vi "FOCUS_V42.vi"(9 "X-pixels":sgl=256.0, 11 "Run":bool) -> (0 "Retrace pixels":sgl, 10 "Pixel Clock (Hz)":sgl)   [LabVIEW 2010] (continued)
            n1000 = Array Max & Min(array=w3024) -> (max value=w3028:dbl, min value=w3027:dbl)  [unwired: 2 out]
            n1001 = Greater?(x=w3028, y=w3021) -> (0:w3026:bool)
            n1002 = Less?(x=w3027, y=w3022) -> (x < y?=w3025:bool)
            n1003 = Or(x=w3026, y=w3025) -> (x .or. y?=w3023:bool)
            n1004 = case shown="False" w3023 {
              tunnel: [u32 16711680 u32 0] -> w3029
              frame True {
              }
              frame False {
                (unwired) u32 16756736
              }
            }
          }
        }
        n1005 = Bundle(w2039, w2040) -> (→"Galvos":cluster{dbl[], dbl[]})  [unwired: 1 in]
        n1006 = local read "frame/line indicator"() -> (w2024:u16)
        n1007 = local read "frame/line indicator"() -> (w1884:u16)
        n1008 = property class="DAQmx Buffer"(reference=w1951, error in=w1949, "Input:Buffer Size"=u32 10000000 ("Input.BufSize")) -> (reference out=w1950:refnum<k21>, error out=w1948:errorcluster)
        n1009 = Concatenate Strings(w1896, tag "/PXI_Trig2" ("source terminal")) -> (w1988:string)
        n1010 = call-poly <vilib>:"DAQmx Create Channel (CO-Pulse Generation-Ticks).vi"("high ticks"=w1876, "low ticks"=w1874, "counter"=w1934, "source of ticks"=w1928, "error in"=w1923, "initial delay"=w1877) -> ("task out"=w1960:refnum<k21>, "error out"=w1959:errorcluster)  [unwired: 8 in]
        n1011 = Greater Or Equal?(x=w2024, y=3.0) -> (x >= y?=w2023:bool)
        n1012 = Concatenate Strings(w1896, tag "/PXI_Trig2" ("destination terminal")) -> (w1992:string)
        n1013 = Bundle("Trigger?"="Trigger?", "Type"="Type", "Level [V]"="Level [V]", "slope"="slope") -> (w1907:T17)  [unwired: 1 in]
        n1014 = Type Cast(type=tag "" ("destination terminal"), x=w1988) -> (*(type *) &x=w1985:tag)
        n1015 = Concatenate Strings(w1896, tag "/10MHzRefClock" ("source terminal")) -> (w1997:string)
        n1016 = Type Cast(type=tag "" ("destination terminal"), x=w1992) -> (*(type *) &x=w1989:tag)
        n1017 = Type Cast(type=tag "" ("destination terminal"), x=w1997) -> (*(type *) &x=w1994:tag)
        n1018 = call-poly <vilib>:"DAQmx Timing (Implicit).vi"("task/channels in"=w1960, "sample mode"=w1958, "error in"=w1959) -> ("task out"=w1957:refnum<k21>, "error out"=w1956:errorcluster)  [unwired: 11 in]
        n1019 = case shown="3" w1884 {
          tunnel: [_ _ w3014 w3017 w3018] -> w2029
          frame 0, Default {
          }
          frame 1 {
          }
          frame 2 {
            n1020 = local read "Y-lines"() -> (w3015:sgl)
            n1021 = local read "Number of frames"() -> (w3016:sgl)
            n1022 = Multiply(x=w3015, y=w3016) -> (x*y=w3014:sgl)
          }
          frame 3 {
            n1023 = local read "Y-lines FreeLine"() -> (w3017:sgl)
          }
          frame 4 {
            n1024 = local read "Y-lines FreeLine"() -> (w3018:sgl)
          }
        }
        n1025 = local read "Fiberscope\nMode"() -> (w1893:bool)
        n1026 = case shown="False" w1893 {
          tunnel: w2023 -> [w2080 _]
          tunnel: w1946 -> [w2079 _]
          tunnel: [w2078 w2083] -> w1915
          frame False {
            n1027 = case shown="False" w2080 {
              tunnel: [w2081 w2082] -> w2078
              tunnel: w2079 -> [_ _]
              frame False {
                n1028 = local read "Pixel Clock (Hz)"() -> (w2081:sgl)
              }
              frame True {
                n1029 = local read "Pixel Clock (Hz) FreeLine"() -> (w2082:sgl)
              }
            }
          }
          frame True {
            n1030 = local read "Pixel Clock (Hz) FScope"() -> (w2083:sgl)
          }
        }
        n1031 = case shown="True" w1916 {
          tunnel: [_ w2977] -> w2013
          tunnel: [_ w2976] -> w2012
          tunnel: w1915 -> [_ w2973]
          tunnel: w1921 -> [_ w2961]
          frame False {
          }
          frame True {
            w2980 = 10123 items=["Finite Samples"=10178, "Continuous Samples"=10123, "Hardware Timed Single Point"=12522] ("sample mode")
            w2981 = 10171 items=["Rising"=10280, "Falling"=10171] ("edge")
            n1032 = local read "AI Device"() -> (w2948:tag)
            n1033 = Concatenate Strings(w2948, tag "/ai0," ("physical channels"), w2948, tag "/ai1," ("physical channels"), w2948, tag "/ai2," ("physical channels"), w2948, tag "/ai3" ("physical channels")) -> (w2970:string)
            n1034 = Type Cast(type=tag "" ("physical channels"), x=w2970) -> (*(type *) &x=w2967:tag)
            n1035 = local read "AO/DIO Device"() -> (w2951:tag)
            n1036 = call-poly <vilib>:"DAQmx Create Channel (AI-Voltage-Basic).vi"("maximum value"=10.0, "physical channels"=w2967, "error in"=w2961) -> ("task out"=w2978:refnum<k21>, "error out"=w2979:errorcluster)  [unwired: 11 in]
            n1037 = Concatenate Strings(tag "/" ("destination terminal"), w2951, tag "/ao/SampleClock" ("source")) -> (w2952:string)
            n1038 = Type Cast(type=tag "" ("source"), x=w2952) -> (*(type *) &x=w2950:tag)
            n1039 = call-poly <vilib>:"DAQmx Timing (Sample Clock).vi"("task/channels in"=w2978, "sample mode"=w2980, "rate"=w2973, "source"=w2950, "error in"=w2979) -> ("task out"=w2960:refnum<k21>, "error out"=w2959:errorcluster)  [unwired: 9 in]
            n1040 = property class="DAQmx Buffer"(reference=w2960, error in=w2959, "Input:Buffer Size"=u32 5000000 ("Input.BufSize")) -> (reference out=w2957:refnum<k21>, error out=w2958:errorcluster)
            n1041 = Concatenate Strings(tag "/" ("destination terminal"), w2951, tag "/ao/StartTrigger" ("source")) -> (w2966:string)
            n1042 = Type Cast(type=tag "" ("source"), x=w2966) -> (*(type *) &x=w2964:tag)
            n1043 = call-poly <vilib>:"DAQmx Start Trigger (Digital Edge).vi"("task/channels in"=w2957, "source"=w2964, "edge"=w2981, "error in"=w2958) -> ("task out"=w2975:refnum<k21>, "error out"=w2974:errorcluster)  [unwired: 10 in]
            n1044 = call <vilib>:"DAQmx Start Task.vi"("task/channels in"=w2975, "error in"=w2974) -> ("task out"=w2977:refnum<k21>, "error out"=w2976:errorcluster)  [unwired: 12 in]
          }
        }
        n1045 = call "AOConfigwriteDAQmx.vi"("AO.UseOnlyOnBrdMem"=FALSE, "TriggerCluster"=w1907, "Trigger Source"=w1906, "Sampling"=w1914, "rate"=w1915, "data"=w1888, "error in"=w1921, "RegenMode"=w2026, "Output.OnbrdBufSize"=w1946, "physical channels"=w2014) -> ("error out"=w2008:errorcluster, "task out"=w2007:refnum<k21>)
        n1046 = call <vilib>:"DAQmx Connect Terminals.vi"("source terminal"=w1994, "destination terminal"=w1989, "error in"=w2008) -> ("error out"=w2027:errorcluster)  [unwired: 12 in]
        n1047 = Concatenate Strings(w1896, tag "/ao/StartTrigger" ("source terminal")) -> (w1899:string)
        n1048 = call <vilib>:"DAQmx Start Task.vi"("task/channels in"=w1957, "error in"=w1956) -> ("task out"=w1955:refnum<k21>, "error out"=w1922:errorcluster)  [unwired: 12 in]
        n1049 = call-poly <vilib>:"DAQmx Timing (Sample Clock).vi"("task/channels in"=w1950, "sample mode"=w2011, "rate"=w1915, "source"=w1963, "error in"=w1948) -> ("task out"=w2010:refnum<k21>, "error out"=w2009:errorcluster)  [unwired: 9 in]
        n1050 = Concatenate Strings(w1896, tag "/PFI2" ("destination terminal")) -> (w1984:string)
        n1051 = Type Cast(type=tag "" ("destination terminal"), x=w1899) -> (*(type *) &x=w1895:tag)
        n1052 = Concatenate Strings(w1896, tag "/PFI5" ("destination terminal")) -> (w1976:string)
        n1053 = Concatenate Strings(w1896, tag "/PFI7" ("destination terminal")) -> (w1905:string)
        n1054 = local read "frame/line indicator"() -> (w2037:u16)
        n1055 = Type Cast(type=tag "" ("destination terminal"), x=w1984) -> (*(type *) &x=w1981:tag)
        n1056 = call <vilib>:"DAQmx Connect Terminals.vi"("source terminal"=w1985, "destination terminal"=w1981, "error in"=w2027) -> ("error out"=w1902:errorcluster)  [unwired: 12 in]
        n1057 = property on="Galvos" class="XYGraph (strict)"("Plot Area:Colors:FG Color"=w2041, "Plot Area:Colors:BG Color"=w2041) -> ()  [unwired: 2 in, 2 out]
        n1058 = Concatenate Strings(w1896, tag "/ao/SampleClock" ("source terminal")) -> (w1980:string)
        n1059 = Type Cast(type=tag "" ("destination terminal"), x=w1976) -> (*(type *) &x=w1973:tag)
        n1060 = Type Cast(type=tag "" ("destination terminal"), x=w1905) -> (*(type *) &x=w1900:tag)
        n1061 = call <vilib>:"DAQmx Connect Terminals.vi"("source terminal"=w1895, "destination terminal"=w1900, "error in"=w1902) -> ("error out"=w1901:errorcluster)  [unwired: 12 in]
        n1062 = call <vilib>:"DAQmx Start Task.vi"("task/channels in"=w2010, "error in"=w2009) -> ("task out"=w2016:refnum<k21>, "error out"=w2015:errorcluster)  [unwired: 12 in]
        n1063 = for {
          N: w2029 -> [_]
          tunnel: [w3019] -> w2030 mode=indexing
          i -> [w3019]
        }
        n1064 = Type Cast(type=tag "" ("destination terminal"), x=w1980) -> (*(type *) &x=w1977:tag)
        n1065 = call <vilib>:"DAQmx Connect Terminals.vi"("source terminal"=w1977, "destination terminal"=w1973, "error in"=w1901) -> ()  [unwired: 12 in, 1 out]
      }
    }
    n1066 = local read "Image3Array"() -> (w170:u8[][])
    n1067 = local read "Image4Array"() -> (w186:u8[][])
    n1068 = local read "Image1Array"() -> (w175:u8[][])
    n1069 = local read "Image2Array"() -> (w185:u8[][])
    n1070 = flat-sequence {
      tunnel: w175 -> [_]
      frame #0 {
        n1071 = property on="Property Node" class="VI"() -> ("VI Path"=w329:path)  [unwired: 2 in, 2 out]
        n1072 = Initialize Array(u8 0 ("x 2")) -> (w314:u8[])  [unwired: 1 in]
        n1073 = Strip Path(path=w329) -> (stripped path=w305:path)  [unwired: 1 out]
        n1074 = local read "VISA Sutter MP-285"() -> (w320:refnum<visa-resource-name>)
        n1075 = local read "MaiTai setting Path"() -> (w316:path)
        n1076 = local read "VISA XPG-ADC"() -> (w318:refnum<visa-resource-name>)
        n1077 = Strip Path(path=w305) -> ()  [unwired: 2 out]
        n1078 = local read "AO/DIO Device"() -> (w333:tag)
        n1079 = local read "AI Device"() -> (w326:tag)
        n1080 = Build Path(base path=w305, name or relative path="FOCUS.cfg") -> (appended path=w309:path)
        n1081 = Path To String(path=w316) -> (string=w315:string)
        n1082 = Type Cast(type="" ("name or relative path"), x=w318) -> (*(type *) &x=w317:string)
        n1083 = Type Cast(type="" ("name or relative path"), x=w320) -> (*(type *) &x=w319:string)
        n1084 = Type Cast(type=w314, x=w326) -> (*(type *) &x=w300:u8[])
        n1085 = Type Cast(type=w314, x=w315) -> (*(type *) &x=w313:u8[])
        n1086 = Type Cast(type=w314, x=w317) -> (*(type *) &x=w323:u8[])
        n1087 = Type Cast(type=w314, x=w319) -> (*(type *) &x=w324:u8[])
        n1088 = Type Cast(type=w314, x=w333) -> (*(type *) &x=w304:u8[])
        n1089 = Array Size(array=w300) -> (size(s)=w301:i32)
        n1090 = Array Size(array=w313) -> (size(s)=w312:i32)
        n1091 = Array Size(array=w304) -> (size(s)=w303:i32)
        n1092 = To Unsigned Byte Integer(number=w301) -> (unsigned 8bit integer=w299:u8)
        n1093 = To Unsigned Byte Integer(number=w312) -> (unsigned 8bit integer=w311:u8)
        n1094 = call <vilib>:"Open_Create_Replace File.vi"("advisory dialog? (display:T)"=FALSE, "function (open:0)"=T8."create or replace", "file path"=w309) -> ("error out"=w307:errorcluster, "refnum"=w308:refnum<file>)  [unwired: 5 in, 2 out]
        n1095 = To Unsigned Byte Integer(number=w303) -> (unsigned 8bit integer=w302:u8)
        n1096 = Build Array (concatenate)(w302, w304, w299, w300, w324, w323, w311, w313) -> (w325:u8[])
        n1097 = Write to Binary File(file (use dialog)=w308, data=w325, error in=w307, 5:FALSE ("prepend array or string size? (T)")) -> (refnum out=w327:refnum<file>, error out=w328:errorcluster)  [unwired: 2 in, 1 out]
        n1098 = Close File(refnum=w327, error in=w328) -> (error out=w331:errorcluster)  [unwired: 1 out]
        n1099 = call <vilib>:"Simple Error Handler.vi"("error in (no error)"=w331) -> ()  [unwired: 4 in, 5 out]
      }
    }
    n1100 = Equal?(x=w181, y=u16 4) -> (x = y?=w179:bool)
    n1101 = local read "ScanLineFreeLine"() -> (w197:sgl[][])
    n1102 = Index Array(array=w197, index (row)=0 ("disabled index (col)")) -> (element=w196:sgl[])  [unwired: 1 in]
    n1103 = Index Array(array=w197, index (row)=1 ("disabled index (col)")) -> (element=w177:sgl[])  [unwired: 1 in]
    n1104 = case shown="False" w179 {
      tunnel: [w334 w338] -> w178
      tunnel: w177 -> [w335 _]
      frame False {
        n1105 = Array Size(array=w335) -> (size(s)=w336:i32)
        n1106 = Initialize Array(sgl 0.0 ("element"), w336) -> (w334:sgl[])
      }
      frame True {
        n1107 = local read "Zsin3D"() -> (w338:sgl[])
      }
    }
    n1108 = Greater Or Equal?(x=w181, y=u16 3) -> (x >= y?=w182:bool)
    n1109 = local write "Ready?"(FALSE ("Ready?")) -> ()
    n1110 = property on="Image 2" class="IntGraph (strict)"() -> ("Color Table"=w288:u32[])  [unwired: 2 in, 2 out]
    n1111 = Interleave 1D Arrays(w196, w177, w178) -> (w192:sgl[])
    n1112 = local read "Positions"() -> (w191:sgl[])
    n1113 = local read "Focus"() -> (w207:bool)
    n1114 = local write "OpenShutter"(FALSE ("OpenShutter")) -> ()
    n1115 = local read "Channel selector"() -> (w159:u8)
    n1116 = Array Size(array=w192) -> (size(s)=w193:i32)
    n1117 = local write "Run"(w207) -> ()
    n1118 = Build Array (concatenate)(w193, w192, w191) -> (w184:sgl[])
    n1119 = flat-sequence {
      tunnel: [w430] -> w295
      tunnel: [w429] -> w162
      tunnel: [w397] -> w291
      tunnel: [w398] -> w290
      tunnel: w288 -> [w408]
      tunnel: w258 -> [w425]
      tunnel: w287 -> [w424]
      tunnel: [w423] -> w286
      tunnel: [w422] -> w285
      tunnel: w282 -> [w421]
      tunnel: w281 -> [w420]
      tunnel: [w399] -> w276
      tunnel: [w400] -> w275
      tunnel: [w386] -> w263
      tunnel: [w403] -> w218
      tunnel: [w402] -> w217
      tunnel: [w401] -> w209
      tunnel: w206 -> [w380]
      tunnel: w170 -> [w379]
      tunnel: w186 -> [w378]
      tunnel: w175 -> [w377]
      tunnel: w185 -> [w376]
      tunnel: w184 -> [w375]
      tunnel: w182 -> [w374]
      tunnel: w167 -> [w362]
      tunnel: [w362] -> w166
      tunnel: [w356] -> w160
      tunnel: w159 -> [w355]
      frame #0 {
        w407 = FALSE ("data")
        w419 = i8 -1 ("element")
        n1120 = local read "Mode selector"() -> (w371:u16)
        n1121 = local read "frame/line indicator"() -> (w427:u16)
        n1122 = local read "ImageSelector"() -> (w416:bool)
        n1123 = Split Number(x=w408) -> (lo(x)=w410:u16[])  [unwired: 1 out]
        n1124 = Split Number(x=w410) -> (lo(x)=w409:u8[])  [unwired: 1 out]
        n1125 = Equal?(x=w427, y=4) -> (x = y?=w361:bool)
        n1126 = Equal?(x=w371, y=4) -> (x = y?=w358:bool)
        n1127 = Or(x=w361, y=w362) -> (x .or. y?=w360:bool)
        n1128 = property on="Intensity" class="Slide (strict)"("Scale.Range:Maximum"="IntensityScaleMax") -> ()  [unwired: 2 in, 2 out]
        n1129 = Not(x=w358) -> (.not. x?=w359:bool)
        n1130 = And(x=w359, y=w360) -> (x .and. y?=w357:bool)
        n1131 = case shown="False" w357 {
          tunnel: [w455 _] -> w395
          tunnel: [w454 _] -> w396
          tunnel: w358 -> [w453 _]
          frame False {
            n1132 = case shown="True" w453 {
              tunnel: [w465 w478] -> w455
              tunnel: [w464 w477] -> w454
              frame False {
                n1133 = local read "AO/DIO Device"() -> (w461:tag)
                n1134 = Concatenate Strings(w461, tag "/ao3" ("physical channels")) -> (w459:string)
                n1135 = Type Cast(type=tag "" ("physical channels"), x=w459) -> (*(type *) &x=w457:tag)
                n1136 = call-poly <vilib>:"DAQmx Create Channel (AO-Voltage-Basic).vi"("physical channels"=w457) -> ("task out"=w462:refnum<k21>, "error out"=w463:errorcluster)  [unwired: 13 in]
                n1137 = local read "Intensity"() -> (w456:sgl)
                n1138 = call-poly <vilib>:"DAQmx Write (Analog DBL 1Chan 1Samp).vi"("task/channels in"=w462, "data"=w456, "error in"=w463) -> ("task out"=w465:refnum<k21>, "error out"=w464:errorcluster)  [unwired: 10 in, 1 out]
              }
              frame True {
                n1139 = local read "AO/DIO Device"() -> (w466:tag)
                n1140 = Concatenate Strings(w466, tag "/ao2," ("physical channels"), w466, tag "/ao3" ("physical channels")) -> (w473:string)
                n1141 = Type Cast(type=tag "" ("physical channels"), x=w473) -> (*(type *) &x=w471:tag)
                n1142 = call-poly <vilib>:"DAQmx Create Channel (AO-Voltage-Basic).vi"("physical channels"=w471) -> ("task out"=w475:refnum<k21>, "error out"=w476:errorcluster)  [unwired: 13 in]
                n1143 = local read "Intensity"() -> (w469:sgl)
                n1144 = Build Array(sgl 0.0 ("element"), w469) -> (w468:sgl[])
                n1145 = call-poly <vilib>:"DAQmx Write (Analog 1D DBL NChan 1Samp).vi"("task/channels in"=w475, "data"=w468, "error in"=w476) -> ("task out"=w478:refnum<k21>, "error out"=w477:errorcluster)  [unwired: 10 in, 1 out]
              }
            }
          }
          frame True {
          }
        }
        n1146 = local read "Fiberscope\nMode"() -> (w401:bool)
        n1147 = call "VISA MP-285 GetSet Speed.vi"("Input: Duty Cluster"=w380, "Input: Speed in microns/sec"="Sutter Speed [um/s]") -> ("Output: Duty Cluster"=w390:T18)  [unwired: 1 out]
        n1148 = call "VISA MP-285 Get Position.vi"("Input: Duty Cluster"=w390) -> ("Output: X axis (microns)"=w382:dbl, "Output: Y axis (microns)"=w383:dbl, "Output: Z axis (microns)"=w388:dbl, "Output: Duty Cluster"=w387:T18)
        n1149 = Multiply(x=w382, y="Sutter scale x") -> (x*y=→"x-positionstart (um)":dbl)
        n1150 = Multiply(x=w383, y="Sutter scale y") -> (x*y=→"y-positionstart (um)":dbl)
        n1151 = local read "frame scan finished?"() -> (w370:bool)
        n1152 = Multiply(x="Sutter scale z", y=w388) -> (x*y=w381:dbl)
        "z-positionstart (um)" <- w381
        n1153 = local read "AO/DIO Device"() -> (w413:tag)
        n1154 = property on="ImageSlide" class="Slide (strict)"() -> ("Scale.Range:Maximum"=w418:dbl, "Visible"=w417:bool)  [unwired: 2 in, 2 out]
        n1155 = case shown="True" w401 {
          tunnel: [_ w447] -> w403
          tunnel: [_ w446] -> w402
          frame False {
          }
          frame True {
            w441 = TRUE ("element")
            n1156 = local read "AO/DIO Device"() -> (w443:tag)
            n1157 = Concatenate Strings(w443, tag "/port2/line6," ("lines"), w443, tag "/port2/line7" ("lines")) -> (w452:string)
            n1158 = Type Cast(type=tag "" ("lines"), x=w452) -> (*(type *) &x=w450:tag)
            n1159 = call-poly <vilib>:"DAQmx Create Channel (DO-Digital Output).vi"("lines"=w450) -> ("task out"=w449:refnum<k21>, "error out"=w448:errorcluster)  [unwired: 13 in]
            n1160 = Build Array(w441, w441) -> (w442:bool[])
            n1161 = call-poly <vilib>:"DAQmx Write (Digital 1D Bool 1Chan 1Samp).vi"("task/channels in"=w449, "data"=w442, "error in"=w448) -> ("task out"=w447:refnum<k21>, "error out"=w446:errorcluster)  [unwired: 10 in, 1 out]
          }
        }
        n1162 = Concatenate Strings(w413, tag "/port1/line1" ("lines")) -> (w415:string)
        n1163 = local read "GetFirst"() -> (w384:bool)
        n1164 = local read "GetLast"() -> (w385:bool)
        n1165 = Type Cast(type=tag "" ("lines"), x=w415) -> (*(type *) &x=w411:tag)
        n1166 = And(x=w370, y="Go back?") -> (x .and. y?=w368:bool)
        n1167 = And(x=w384, y=w385) -> (x .and. y?=w373:bool)
        n1168 = call-poly <vilib>:"DAQmx Create Channel (DO-Digital Output).vi"("lines"=w411) -> ("task out"=w406:refnum<k21>, "error out"=w405:errorcluster)  [unwired: 13 in]
        "Shutter" <- w406
        n1169 = Or(x=w368, y=w373) -> (x .or. y?=w366:bool)
        n1170 = case shown="True" w366 {
          tunnel: w387 -> [w432 w440]
          tunnel: [w432 w439] -> w386
          tunnel: w381 -> [_ w437]
          tunnel: [FALSE ("IntDevUsed 2") FALSE ("IntDevUsed 2")] -> w367
          frame False {
          }
          frame True {
            n1171 = local read "FirstPosition"() -> (w436:sgl)
            n1172 = local read "Sutter scale z"() -> (w433:sgl)
            n1173 = Subtract(x=w436, y=w437) -> (x-y=w435:dbl)
            n1174 = Divide(x=w435, y=w433) -> (x/y=w438:dbl)
            n1175 = call "VISA MP-285 Step.vi"("Input: Duty Cluster"=w440, "Input: Delta Z axis (microns)"=w438) -> ("Output: Duty Cluster"=w439:T18)  [unwired: 2 in, 3 out]
          }
        }
        n1176 = local write "frame scan finished?"(w367) -> ()
        n1177 = local write "Shutter open"(w407) -> ()
        n1178 = call-poly <vilib>:"DAQmx Write (Digital Bool 1Line 1Point).vi"("task/channels in"=w406, "data"=w407, "error in"=w405) -> ("task out"=w393:refnum<k21>, "error out"=w394:errorcluster)  [unwired: 10 in, 1 out]
        n1179 = while {
          tunnel: ["Run"] -> w430
          tunnel: ["End experiment"] -> w429
          shift-right: [w580] -> _
          shift-left: w408 -> [w583]
          shift-right: [w578] -> _
          shift-left: FALSE ("Visible") -> [w579]
          tunnel: w425 -> [w577]
          tunnel: w424 -> [w576]
          tunnel: [w577] -> w423
          tunnel: [w576] -> w422
          tunnel: w421 -> [w574]
          tunnel: w420 -> [w566]
          shift-right: [w539] -> _
          shift-left: w419 -> [w540]
          shift-right: [w537] -> _
          shift-left: w419 -> [w538]
          tunnel: w418 -> [w536]
          tunnel: w417 -> [w535]
          shift-right: [w528] -> _
          shift-left: w416 -> [w527]
          shift-right: [w521] -> _
          shift-left: w409 -> [w522]
          tunnel: [w501] -> w400
          tunnel: [w500] -> w399
          tunnel: [w505] -> w398
          tunnel: [w504] -> w397
          tunnel: w396 -> [w507]
          tunnel: w395 -> [w506]
          tunnel: w394 -> [w503]
          tunnel: w393 -> [w502]
          tunnel: w379 -> [w487]
          tunnel: w378 -> [w486]
          tunnel: w377 -> [w488]
          tunnel: w376 -> [w489]
          tunnel: w375 -> [w492]
          tunnel: w374 -> [w490]
          tunnel: [w480] -> w356
          shift-right: [w479] -> _
          shift-left: w355 -> [w481]
          i -> [w526]
          stop <- w517 stop-if-true
          n1180 = local read "index (row)1"() -> (w545:i32)
          n1181 = property on="Image 2" class="IntGraph (strict)"() -> ("Color Table"=w582:u32[])  [unwired: 2 in, 2 out]
          n1182 = event shown="[0] Timeout" {
            selector: _ -> [_ _ _ _ _ _ _ _ _ _ _ _ _ _ _ _ _ _ _ _ _ _ _ _ _ _ _ _ _ _ _ _ _ _ _]
            dyn-events: _ -> [_ _ _ _ _ _ _ _ _ _ _ _ _ _ _ _ _ _ _ _ _ _ _ _ _ _ _ _ _ _ _ _ _ _ _]
            timeout: 0 -> [_ _ _ _ _ _ _ _ _ _ _ _ _ _ _ _ _ _ _ _ _ _ _ _ _ _ _ _ _ _ _ _ _ _ _]
            tunnel: [FALSE ("Fiberscope\nMode") TRUE ("Fiberscope\nMode") TRUE ("Fiberscope\nMode") TRUE ("Fiberscope\nMode") TRUE ("Fiberscope\nMode") TRUE ("Fiberscope\nMode") TRUE ("Fiberscope\nMode") TRUE ("Fiberscope\nMode") TRUE ("Fiberscope\nMode") TRUE ("Fiberscope\nMode") TRUE ("Fiberscope\nMode") TRUE ("Fiberscope\nMode") TRUE ("Fiberscope\nMode") TRUE ("Fiberscope\nMode") TRUE ("Fiberscope\nMode") TRUE ("Fiberscope\nMode") TRUE ("Fiberscope\nMode") TRUE ("Fiberscope\nMode") TRUE ("Fiberscope\nMode") TRUE ("Fiberscope\nMode") TRUE ("Fiberscope\nMode") TRUE ("Fiberscope\nMode") TRUE ("Fiberscope\nMode") TRUE ("Fiberscope\nMode") TRUE ("Fiberscope\nMode") TRUE ("Fiberscope\nMode") TRUE ("Fiberscope\nMode") TRUE ("Fiberscope\nMode") TRUE ("Fiberscope\nMode") FALSE ("Fiberscope\nMode") _ FALSE ("Fiberscope\nMode") FALSE ("Fiberscope\nMode") FALSE ("Fiberscope\nMode") FALSE ("Fiberscope\nMode")] -> w509
            tunnel: [_ _ _ _ _ _ _ _ w656 _ _ _ _ _ _ _ _ _ _ _ _ _ _ _ _ _ _ _ _ _ _ _ _ _ _] -> w508
            tunnel: w507 -> [w614 w619 w624 w629 w634 w639 w644 w649 w654 w660 w665 w670 w675 w680 w685 w690 w695 w700 w705 w710 w715 w720 w725 w730 w735 w740 w745 w750 w756 w764 w769 w776 w796 w801 w808]
            tunnel: w506 -> [w615 w620 w625 w630 w635 w640 w645 w650 w655 w661 w666 w671 w676 w681 w686 w691 w696 w701 w706 w711 w716 w721 w726 w731 w736 w741 w746 w751 w757 w763 w770 w777 w797 w802 w809]
            tunnel: [w614 w619 w624 w629 w634 w639 w644 w649 w654 w660 w665 w670 w675 w680 w685 w690 w695 w700 w705 w710 w715 w720 w725 w730 w735 w740 w745 w750 w756 w762 w769 w776 w796 w801 w808] -> w505
            tunnel: [w615 w620 w625 w630 w635 w640 w645 w650 w655 w661 w666 w671 w676 w681 w686 w691 w696 w701 w706 w711 w716 w721 w726 w731 w736 w741 w746 w751 w757 w761 w770 w777 w797 w802 w809] -> w504
            tunnel: w503 -> [w612 w617 w622 w627 w632 w637 w642 w647 w652 w658 w663 w668 w673 w678 w683 w688 w693 w698 w703 w708 w713 w718 w723 w728 w733 w738 w743 w748 w754 w759 w773 w774 w794 w799 w806]
            tunnel: w502 -> [w613 w618 w623 w628 w633 w638 w643 w648 w653 w659 w664 w669 w674 w679 w684 w689 w694 w699 w704 w709 w714 w719 w724 w729 w734 w739 w744 w749 w755 w760 w772 w775 w795 w800 w807]
            tunnel: [w612 w617 w622 w627 w632 w637 w642 w647 w652 w658 w663 w668 w673 w678 w683 w688 w693 w698 w703 w708 w713 w718 w723 w728 w733 w738 w743 w748 w754 w759 w768 w774 w794 w799 w806] -> w501
            tunnel: [w613 w618 w623 w628 w633 w638 w643 w648 w653 w659 w664 w669 w674 w679 w684 w689 w694 w699 w704 w709 w714 w719 w724 w729 w734 w739 w744 w749 w755 w760 w767 w775 w795 w800 w807] -> w500
            tunnel: w492 -> [_ _ _ _ _ _ _ _ _ _ _ _ _ _ _ _ _ _ _ _ _ _ _ _ _ _ _ _ _ _ _ _ w790 _ _]
            tunnel: w490 -> [_ _ _ _ _ _ _ _ _ _ _ _ _ _ _ _ _ _ _ _ _ _ _ _ _ _ _ _ _ _ _ _ w786 _ _]
            tunnel: w488 -> [_ _ _ _ _ _ _ _ _ _ _ _ _ _ _ _ _ _ _ _ _ _ _ _ _ _ _ _ _ _ _ _ _ _ _]
            tunnel: w489 -> [_ _ _ _ _ _ _ _ _ _ _ _ _ _ _ _ _ _ _ _ _ _ _ _ _ _ _ _ _ _ _ _ _ _ _]
            tunnel: w487 -> [_ _ _ _ _ _ _ _ _ _ _ _ _ _ _ _ _ _ _ _ _ _ _ _ _ _ _ _ _ _ _ _ _ _ _]
            tunnel: w486 -> [_ _ _ _ _ _ _ _ _ _ _ _ _ _ _ _ _ _ _ _ _ _ _ _ _ _ _ _ _ _ _ _ _ _ _]
            event Timeout {
              n1183 = event-data() -> ()  [unwired: 1 in, 2 out]
            }
            event "Mode selector": Value Change {
              n1184 = event-data() -> ()  [unwired: 1 in, 2 out]
            }
            event "Scan format": Value Change {
              n1185 = event-data() -> ()  [unwired: 1 in, 2 out]
            }
            event "Measurement cursor check box": Value Change {
              n1186 = event-data() -> ()  [unwired: 1 in, 2 out]
            }
            event "View line\ncheck box": Value Change {
              n1187 = event-data() -> ()  [unwired: 1 in, 2 out]
            }
            event "X-pixels": Value Change {
              n1188 = event-data() -> ()  [unwired: 1 in, 2 out]
            }
            event "Y-lines": Value Change {
              n1189 = event-data() -> ()  [unwired: 1 in, 2 out]
            }
            event "line scan time (ms)": Value Change {
              n1190 = event-data() -> ()  [unwired: 1 in, 2 out]
            }
            event "Type": Value Change {
              n1191 = event-data() -> ("NewVal"=w656:bool)  [unwired: 1 in, 1 out]
            }
            event "Level [V]": Value Change {
              n1192 = event-data() -> ()  [unwired: 1 in, 2 out]
            }
            event "Number of stacks": Value Change {
              n1193 = event-data() -> ()  [unwired: 1 in, 2 out]
            }
            event "new FreeLine?": Value Change {
              n1194 = event-data() -> ()  [unwired: 1 in, 2 out]
            }
            event "FocusModeSelector": Value Change {
              n1195 = event-data() -> ()  [unwired: 1 in, 2 out]
            }
            event "Trigger?": Value Change {
              n1196 = event-data() -> ()  [unwired: 1 in, 2 out]
            }
            event "Number of frames": Value Change {
              n1197 = event-data() -> ()  [unwired: 1 in, 2 out]
            }
            event "Averaging": Value Change {
              n1198 = event-data() -> ()  [unwired: 1 in, 2 out]
            }
            event "z-step (um)": Value Change {
              n1199 = event-data() -> ()  [unwired: 1 in, 2 out]
            }
            event "Fiberscope\nMode": Value Change {
              n1200 = event-data() -> ()  [unwired: 1 in, 3 out]
            }
            event "NewScanpattern": Value Change {
              n1201 = event-data() -> ()  [unwired: 1 in, 3 out]
            }
            event "Scan format FScope": Value Change {
              n1202 = event-data() -> ()  [unwired: 1 in, 3 out]
            }
            event "X dim": Value Change {
              n1203 = event-data() -> ()  [unwired: 1 in, 3 out]
            }
            event "Y dim": Value Change {
              n1204 = event-data() -> ()  [unwired: 1 in, 3 out]
            }
            event "Mode selectorFScope": Value Change {
              n1205 = event-data() -> ()  [unwired: 1 in, 3 out]
            }
            event "Number of Frames": Value Change {
              n1206 = event-data() -> ()  [unwired: 1 in, 3 out]
            }
            event "Averaging": Value Change {
              n1207 = event-data() -> ()  [unwired: 1 in, 3 out]
            }
            event "LS X/Y": Value Change {
              n1208 = event-data() -> ()  [unwired: 1 in, 3 out]
            }
            event "Number of Stacks": Value Change {
              n1209 = event-data() -> ()  [unwired: 1 in, 3 out]
            }
            event "Time interval [s]": Value Change {
              n1210 = event-data() -> ()  [unwired: 1 in, 3 out]
            }
            event "Scanpattern": Value Change {
              n1211 = event-data() -> ()  [unwired: 1 in, 3 out]
            }
            event "Intensity": Value Change {
              n1212 = event-data() -> ()  [unwired: 1 in, 2 out]
              n1213 = local read "Intensity"() -> (w758:sgl)
              n1214 = call-poly <vilib>:"DAQmx Write (Analog DBL 1Chan 1Samp).vi"("task/channels in"=w763, "data"=w758, "error in"=w764) -> ("task out"=w761:refnum<k21>, "error out"=w762:errorcluster)  [unwired: 10 in, 1 out]
              n1215 = Build Array(sgl 0.0 ("value"), w758) -> ()  [unwired: 1 out]
            }
            event "OpenShutter": Value Change {
              n1216 = event-data() -> ()  [unwired: 1 in, 2 out]
              n1217 = call-poly <vilib>:"DAQmx Write (Digital Bool 1Line 1Point).vi"("task/channels in"=w772, "data"="OpenShutter", "error in"=w773) -> ("task out"=w767:refnum<k21>, "error out"=w768:errorcluster)  [unwired: 10 in, 1 out]
              n1218 = local write "Shutter open"("OpenShutter") -> ()
            }
            event "2Ch\noverlay\nbutton": Mouse Down {
              n1219 = event-data() -> ()  [unwired: 1 in, 2 out]
              n1220 = call "OverlayFOCUS.vi"() -> ()  [unwired: 1 in]
            }
            event "Save? 2": Value Change {
              n1221 = event-data() -> ()  [unwired: 1 in, 1 out]
              n1222 = property on="Property Node" class="VI"() -> ("VI Path"=w783:path)  [unwired: 2 in, 2 out]
              n1223 = local read "FilePath"() -> (w788:path)
              n1224 = local read "NotebookFile"() -> (w780:path)
              n1225 = local read "Header"() -> (w784:u8[])
              n1226 = local read "BaseFilename"() -> (w789:string)
              n1227 = Bundle("BaseFilename"=w789, "FilePath"=w788, "Autoincrement Filename"="Autoincrement Filename", w786) -> (w785:T19)  [unwired: 1 in]
              n1228 = call "SavenewFOCUS.vi"("source path"=w783, "Header"=w784, "Positions"=w790, "Parameters"=w785) -> ("Data directory out"=w779:path, "name"=→"Filename":string, "basename out"=w792:string)
              n1229 = local write "BaseFilename"(w792) -> ()
              n1230 = local write "FilePath"(w779) -> ()
              n1231 = call "SaveNotebookFOCUS.vi"("Notebook Window"="Notebook Window", "NotebookFile"=w780, "FilePathCurrent"=w779) -> ("NotebookFile"=w782:path)
              n1232 = local write "NotebookFile"(w782) -> ()
              "Save?" <- TRUE ("Save?")
            }
            event "Different Integrator Setting": Mouse Down {
              n1233 = event-data() -> ()  [unwired: 1 in, 1 out]
              n1234 = call "IntegratorSetting.vi"("VISA resource name"="VISA XPG-ADC") -> ()
            }
            event "MaiTai setting": Mouse Down {
              n1235 = event-data() -> ()  [unwired: 1 in, 1 out]
              n1236 = call "RunAppl.vi"("Path"="MaiTai setting Path") -> ()
            }
          }
          n1237 = local read "Channel selector"() -> (w479:u8)
          n1238 = Subtract(x=w545, y="SlideHorizontal") -> (x-y=w544:u32)
          n1239 = case shown="False" "Different colour table" {
            tunnel: [w1415 w1432] -> w514
            tunnel: "Default colour table" -> [w1416 _]
            tunnel: w583 -> [w1414 w1434]
            tunnel: "reset?" -> [_ w1440]
            tunnel: w582 -> [w1413 _]
            tunnel: [w1412 w1433] -> w580
            tunnel: w579 -> [w1411 w1438]
            tunnel: [w1410 w1437] -> w578
            tunnel: [w1408 w1431] -> w521
            tunnel: w522 -> [w1409 w1428]
            tunnel: [w1406 w1427] -> w483
            tunnel: [w1407 w1426] -> w484
            frame False {
              n1240 = case shown="True" w1416 {
                tunnel: [w1420 w1421] -> w1415
                tunnel: w1414 -> [w1419 _]
                tunnel: w1413 -> [w1420 _]
                tunnel: [w1419 w1421] -> w1412
                tunnel: w1411 -> [w1418 w1423]
                tunnel: [w1418 w1423] -> w1410
                tunnel: w1409 -> [w1417 _]
                tunnel: [w1417 u8[] [255, 0, 1, 2, 3, 4, 5, 6, 7, 8, 9, 10, 11, 12, 13, 14, 15, 16, 17, 18, 19, 20, 21, 22, 23, 24, 25, 26, 27, 28, 29, 30, 31, 32, 33, 34, 35, 36, 37, 38, 39, 40, 41, 42, 43, 44, 45, 46, 47, 48, 49, 50, 51, 52, 53, 54, 55, 56, 57, 58, 59, 60, 61, 62, 64, 65, 66, 67, 68, 69, 70, 71, 72, 73, 74, 75, 76, 77, 78, 79, 80, 81, 82, 83, 84, 85, 86, 87, 88, 89, 90, 91, 92, 93, 94, 95, 96, 97, 98, 99, 100, 101, 102, 103, 104, 105, 106, 107, 108, 109, 110, 111, 112, 113, 114, 115, 116, 117, 118, 119, 120, 121, 122, 123, 124, 125, 126, 127, 128, 129, 130, 131, 132, 133, 134, 135, 136, 137, 138, 139, 140, 141, 142, 143, 144, 145, 146, 147, 148, 149, 150, 151, 152, 153, 154, 155, 156, 157, 158, 159, 160, 161, 162, 163, 164, 165, 166, 167, 168, 169, 170, 171, 172, 173, 174, 175, 176, 177, 178, 179, 180, 181, 182, 183, 184, 185, 186, 187, 188, 189, 191, 192, 193, 194, 195, 196, 197, 198, 199, 200, 201, 202, 203, 204, 205, 206, 207, 208, 209, 210, 211, 212, 213, 214, 215, 216, 217, 218, 219, 220, 221, 222, 223, 224, 225, 226, 227, 228, 229, 230, 231, 232, 233, 234, 235, 236, 237, 238, 239, 240, 241, 242, 243, 244, 245, 246, 247, 248, 249, 250, 251, 252, 253, 254, 255, 0] ("ColorFactor")] -> w1408
                frame False {
                }
                frame True {
                  w1421 = u32[] [255, 0, 65793, 131586, 197379, 263172, 328965, 394758, 460551, 526344, 592137, 657930, 723723, 789516, 855309, 921102, 986895, 1052688, 1118481, 1184274, 1250067, 1315860, 1381653, 1447446, 1513239, 1579032, 1644825, 1710618, 1776411, 1842204, 1907997, 1973790, 2039583, 2105376, 2171169, 2236962, 2302755, 2368548, 2434341, 2500134, 2565927, 2631720, 2697513, 2763306, 2829099, 2894892, 2960685, 3026478, 3092271, 3158064, 3223857, 3289650, 3355443, 3421236, 3487029, 3552822, 3618615, 3684408, 3750201, 3815994, 3881787, 3947580, 4013373, 4079166, 4210752, 4276545, 4342338, 4408131, 4473924, 4539717, 4605510, 4671303, 4737096, 4802889, 4868682, 4934475, 5000268, 5066061, 5131854, 5197647, 5263440, 5329233, 5395026, 5460819, 5526612, 5592405, 5658198, 5723991, 5789784, 5855577, 5921370, 5987163, 6052956, 6118749, 6184542, 6250335, 6316128, 6381921, 6447714, 6513507, 6579300, 6645093, 6710886, 6776679, 6842472, 6908265, 6974058, 7039851, 7105644, 7171437, 7237230, 7303023, 7368816, 7434609, 7500402, 7566195, 7631988, 7697781, 7763574, 7829367, 7895160, 7960953, 8026746, 8092539, 8158332, 8224125, 8289918, 8355711, 8421504, 8487297, 8553090, 8618883, 8684676, 8750469, 8816262, 8882055, 8947848, 9013641, 9079434, 9145227, 9211020, 9276813, 9342606, 9408399, 9474192, 9539985, 9605778, 9671571, 9737364, 9803157, 9868950, 9934743, 10000536, 10066329, 10132122, 10197915, 10263708, 10329501, 10395294, 10461087, 10526880, 10592673, 10658466, 10724259, 10790052, 10855845, 10921638, 10987431, 11053224, 11119017, 11184810, 11250603, 11316396, 11382189, 11447982, 11513775, 11579568, 11645361, 11711154, 11776947, 11842740, 11908533, 11974326, 12040119, 12105912, 12171705, 12237498, 12303291, 12369084, 12434877, 12566463, 12632256, 12698049, 12763842, 12829635, 12895428, 12961221, 13027014, 13092807, 13158600, 13224393, 13290186, 13355979, 13421772, 13487565, 13553358, 13619151, 13684944, 13750737, 13816530, 13882323, 13948116, 14013909, 14079702, 14145495, 14211288, 14277081, 14342874, 14408667, 14474460, 14540253, 14606046, 14671839, 14737632, 14803425, 14869218, 14935011, 15000804, 15066597, 15132390, 15198183, 15263976, 15329769, 15395562, 15461355, 15527148, 15592941, 15658734, 15724527, 15790320, 15856113, 15921906, 15987699, 16053492, 16119285, 16185078, 16250871, 16316664, 16382457, 16448250, 16514043, 16579836, 16645629, 16711422, 16777215, 16711680] ("Array")
                  n1241 = local write "Default colour table"(FALSE ("Visible")) -> ()
                  n1242 = local write "reset?"(125.0 ("element")) -> ()
                  n1243 = property on="Image 2" class="IntGraph (strict)"("Color Table"=w1421) -> ()  [unwired: 2 in, 2 out]
                  n1244 = property on="Image 1" class="IntGraph (strict)"("Color Table"=w1421) -> ()  [unwired: 2 in, 2 out]
                }
              }
              n1245 = local read "CT1"() -> (w1407:bool)
              n1246 = local read "CT2"() -> (w1406:bool)
            }
            frame True {
              n1247 = local read "Image 1"() -> (w1430:u8[][])
              n1248 = local read "Image 2"() -> (w1429:u8[][])
              n1249 = call "ColorTableGeneratorBWCLFOCUS.vi"("ColourFactor"=w1428, "Image 2"=w1429, "Stop?"=w1438, "Reset"=w1440, "old colour table"=w1434, "Image 1"=w1430) -> ("ColourFactor"=w1431:u32[], "New ClTb"=w1436:bool, 2:w1435:u32[], "Stop?"=w1437:bool, "Ch2"=w1427:bool, "Ch1"=w1426:bool)
              n1250 = local write "Different colour table"(w1437) -> ()
              n1251 = local write "reset?"(0.0 ("element")) -> ()
              n1252 = case shown="True" w1436 {
                tunnel: w1435 -> [w1442 w1443]
                tunnel: [w1442 w1443] -> w1432
                tunnel: [w1441 w1443] -> w1433
                tunnel: w1434 -> [w1441 _]
                frame False {
                }
                frame True {
                }
              }
            }
          }
          "CT2" <- w483
          "CT1" <- w484
          n1253 = local read "Average1"() -> (w556:i32)
          n1254 = property on="Image 3" class="IntGraph (strict)"("Active Cursor"=u32 0, "Cursor.Visible"=TRUE, "Cursor.Cursor Color"=u32 16711680, "Cursor.Cursor Position:Cursor X"=w544, "Cursor.Cursor Position:Cursor Y"=i8 -1 ("Active Cursor")) -> ()  [unwired: 2 in, 2 out]
          n1255 = Not Equal?(x=w481, y=w479) -> (x != y?=w480:bool)
          n1256 = Add(x=w544, y=w556) -> (x+y=w565:u32)
          n1257 = property on="Image 3" class="IntGraph (strict)"("Active Cursor"=u32 1, "Cursor.Visible"=TRUE, "Cursor.Cursor Color"=u32 16711680, "Cursor.Cursor Position:Cursor X"=w565, "Cursor.Cursor Position:Cursor Y"=i8 -1 ("Active Cursor")) -> ()  [unwired: 2 in, 2 out]
          n1258 = property on="Level [V]" class="DigNum (strict)"("Visible"=w508) -> ()  [unwired: 2 in, 2 out]
          n1259 = local read "index (row)2"() -> (w542:i32)
          n1260 = local read "frame/line indicator"() -> (w524:u16)
          n1261 = local read "Overlay Images"() -> (w575:bool)
          n1262 = Compound Arithmetic op=OR("Run", w509, "Open?", "End experiment", "Focus", w480) -> (w517:bool)
          n1263 = case shown="True" "Focus" {
            frame False {
            }
            frame True {
              w811 = u16 0 items=["Focus mode", "Frame scan", "Straight line scan", "FreeLine 2D", "Frame scan piezo", "FreeLine 3D"] ("Mode selector")
              n1264 = local write "Mode selector"(w811) -> ()
            }
          }
          n1265 = Subtract(x=w542, y="SlideHorizontal") -> (x-y=w541:u32)
          n1266 = Not Or(1:w483, 2:w484) -> (0:w482:bool)
          n1267 = Equal?(x=w524, y=u16 3) -> (x = y?=w532:bool)
          n1268 = And(x=w484, y=w483) -> (x .and. y?=w485:bool)
          n1269 = local read "Average2"() -> (w555:i32)
          n1270 = case shown="False" w482 {
            tunnel: w575 -> [w590 _]
            tunnel: w521 -> [w589 _]
            tunnel: w514 -> [w588 _]
            tunnel: w485 -> [w587 _]
            tunnel: w484 -> [w586 _]
            frame False {
              n1271 = case shown="False" w590 {
                tunnel: w588 -> [w594 _]
                tunnel: w589 -> [_ w603]
                tunnel: w587 -> [w593 _]
                tunnel: w586 -> [w592 _]
                frame False {
                  w591 = FALSE ("CT1")
                  n1272 = case shown="False" w593 {
                    tunnel: w594 -> [w596 w598]
                    tunnel: w592 -> [_ w597]
                    frame True {
                      n1273 = property on="Image 2" class="IntGraph (strict)"("Color Table"=w596) -> ()  [unwired: 2 in, 2 out]
                      n1274 = property on="Image 1" class="IntGraph (strict)"("Color Table"=w596) -> ()  [unwired: 2 in, 2 out]
                      "colour table" <- w596
                    }
                    frame False {
                      n1275 = case shown="False" w597 {
                        tunnel: w598 -> [w599 w600]
                        frame False {
                          n1276 = property on="Image 2" class="IntGraph (strict)"("Color Table"=w599) -> ()  [unwired: 2 in, 2 out]
                          "colour table 2" <- w599
                        }
                        frame True {
                          n1277 = local write "colour table"(w600) -> ()
                          n1278 = property on="Image 1" class="IntGraph (strict)"("Color Table"=w600) -> ()  [unwired: 2 in, 2 out]
                        }
                      }
                    }
                  }
                  n1279 = local write "CT1"(w591) -> ()
                  n1280 = local write "CT2"(w591) -> ()
                  n1281 = property on="Image 2" class="IntGraph (strict)"("Visible"=TRUE) -> ()  [unwired: 2 in, 2 out]
                }
                frame True {
                  n1282 = call "ColourFactor.vi"("ColorFactor"=w603, "ColorTable"=u32[] [255, 327680, 328192, 328960, 132352, 1280, 655360, 656640, 657920, 330240, 2560, 983040, 985088, 986880, 528128, 3840, 1310720, 1313280, 1315840, 660480, 5120, 1638400, 1641472, 1644800, 792832, 6400, 1966080, 1969920, 1973760, 990720, 7680, 2293760, 2298368, 2302720, 1188608, 8960, 2621440, 2626560, 2631680, 1320960, 10240, 2949120, 2954752, 2960640, 1453312, 11520, 3276800, 3283200, 3289600, 1651200, 12800, 3604480, 3611648, 3618560, 1849088, 14080, 3932160, 3939840, 3947520, 1981440, 15360, 4259840, 4268032, 4276480, 2113792, 16640, 4587520, 4596480, 4605440, 2311680, 17920, 4915200, 4924928, 4934400, 2509568, 19200, 5242880, 5253120, 5263360, 2641920, 20480, 5570560, 5581312, 5592320, 2774272, 21760, 5898240, 5909760, 5921280, 2972160, 23040, 6225920, 6238208, 6250240, 3170048, 24320, 6553600, 6566400, 6579200, 3302400, 25600, 6881280, 6894592, 6908160, 3434752, 26880, 7208960, 7223040, 7237120, 3632640, 28160, 7536640, 7551488, 7566080, 3830528, 29440, 7864320, 7879680, 7895040, 3962880, 30720, 8192000, 8207872, 8224000, 4095232, 32000, 8519680, 8536320, 8552960, 4293120, 33280, 8847360, 8864768, 8881920, 4491008, 34560, 9175040, 9192960, 9210880, 4623360, 35840, 9502720, 9521152, 9539840, 4755712, 37120, 9830400, 9849600, 9868800, 4953600, 38400, 10158080, 10178048, 10197760, 5151488, 39680, 10485760, 10506240, 10526720, 5283840, 40960, 10813440, 10834432, 10855680, 5416192, 42240, 11141120, 11162880, 11184640, 5614080, 43520, 11468800, 11491328, 11513600, 5811968, 44800, 11796480, 11819520, 11842560, 5944320, 46080, 12124160, 12147712, 12171520, 6076672, 47360, 12451840, 12476160, 12500480, 6274560, 48640, 12779520, 12804608, 12829440, 6472448, 49920, 13107200, 13132800, 13158400, 6604800, 51200, 13434880, 13460992, 13487360, 6737152, 52480, 13762560, 13789440, 13816320, 6935040, 53760, 14090240, 14117888, 14145280, 7132928, 55040, 14417920, 14446080, 14474240, 7265280, 56320, 14745600, 14774272, 14803200, 7397632, 57600, 15073280, 15102720, 15132160, 7595520, 58880, 15400960, 15431168, 15461120, 7793408, 60160, 15728640, 15759360, 15790080, 7925760, 61440, 16056320, 16087552, 16119040, 8058112, 62720, 16384000, 16416000, 16448000, 8256000, 64000, 16763080, 16768200, 16777215, 14483400, 13172680] ("Array")) -> ("ColorTable"=w602:u32[])
                  n1283 = local write "colour table"(w602) -> ()
                  n1284 = property on="Image 2" class="IntGraph (strict)"("Visible"=FALSE) -> ()  [unwired: 2 in, 2 out]
                  n1285 = property on="Image 1" class="IntGraph (strict)"("Color Table"=w602) -> ()  [unwired: 2 in, 2 out]
                }
              }
            }
            frame True {
            }
          }
          n1286 = Equal?(x=w524, y=u16 4) -> (x = y?=w523:bool)
          n1287 = case shown="False" "ImageSelector" {
            selector: "ImageSelector" -> [w830 w841]
            tunnel: w536 -> [_ w839]
            tunnel: w535 -> [_ w840]
            tunnel: [w828 w840] -> w534
            tunnel: [w827 w839] -> w530
            tunnel: w532 -> [w826 _]
            tunnel: w523 -> [w825 _]
            frame False {
              n1288 = property on="Image 3" class="IntGraph (strict)"("Visible"=w830) -> ()  [unwired: 2 in, 2 out]
              n1289 = property on="Histogram1" class="XYGraph (strict)"("Visible"=w830) -> ()  [unwired: 2 in, 2 out]
              n1290 = property on="Image 4" class="IntGraph (strict)"("Visible"=w830) -> ()  [unwired: 2 in, 2 out]
              n1291 = property on="Histogram2" class="XYGraph (strict)"("Visible"=w830) -> ()  [unwired: 2 in, 2 out]
              n1292 = case shown="False" w826 {
                tunnel: [w832 sgl 0.0] -> w827
                tunnel: w825 -> [w831 _]
                frame False {
                  n1293 = case shown="False" w831 {
                    tunnel: [w833 w834] -> w832
                    frame False {
                      n1294 = local read "ImageSlideMax"() -> (w833:sgl)
                    }
                    frame True {
                      n1295 = local read "Number of frames"() -> (w835:sgl)
                      n1296 = Decrement(x=w835) -> (x-1=w834:sgl)
                    }
                  }
                }
                frame True {
                }
              }
              n1297 = Less Or Equal To 0?(x=w827) -> (x <= 0?=w829:bool)
              n1298 = case shown="False" w829 {
                tunnel: [TRUE ("Visible") FALSE ("Visible")] -> w828
                frame False {
                }
                frame True {
                }
              }
            }
            frame True {
              n1299 = property on="Image 3" class="IntGraph (strict)"("Visible"=w841) -> ()  [unwired: 2 in, 2 out]
              n1300 = property on="Histogram1" class="XYGraph (strict)"("Visible"=w841) -> ()  [unwired: 2 in, 2 out]
              n1301 = property on="Image 4" class="IntGraph (strict)"("Visible"=w841) -> ()  [unwired: 2 in, 2 out]
              n1302 = property on="Histogram2" class="XYGraph (strict)"("Visible"=w841) -> ()  [unwired: 2 in, 2 out]
            }
          }
          n1303 = case shown="False" "XScale" {
            tunnel: [w819 w824] -> w568
            tunnel: [w821 0.0 ("Scale.Range:Minimum")] -> w570
            tunnel: [TRUE ("Ready?") FALSE ("Ready?")] -> w569
            frame False {
              n1304 = local read "X-pixels FreeLine"() -> (w820:sgl)
              n1305 = local read "Y-lines FreeLine"() -> (w819:sgl)
              n1306 = Subtract(x=w820, y=w819) -> (x-y=w821:sgl)
            }
            frame True {
              n1307 = local read "X-pixels FreeLine"() -> (w824:sgl)
            }
          }
          n1308 = property on="Image 4" class="IntGraph (strict)"("Active Cursor"=u32 0, "Cursor.Visible"=TRUE, "Cursor.Cursor Color"=u32 16711680, "Cursor.Cursor Position:Cursor X"=w541, "Cursor.Cursor Position:Cursor Y"=i8 -1 ("Active Cursor")) -> ()  [unwired: 2 in, 2 out]
          n1309 = Add(x=w541, y=w555) -> (x+y=w546:u32)
          n1310 = Not Equal?(x=w527, y="ImageSelector") -> (x != y?=w519:bool)
          n1311 = property on="Image 4" class="IntGraph (strict)"("Active Cursor"=u32 1, "Cursor.Visible"=TRUE, "Cursor.Cursor Color"=u32 16711680, "Cursor.Cursor Position:Cursor X"=w546, "Cursor.Cursor Position:Cursor Y"=i8 -1 ("Active Cursor")) -> ()  [unwired: 2 in, 2 out]
          n1312 = property on="Image 3" class="IntGraph (strict)"("X Scale.Range:Maximum"=w568) -> ()  [unwired: 2 in, 2 out]
          n1313 = local read "Mode selector"() -> (w497:u16)
          n1314 = property on="SlideHorizontal" class="Slide (strict)"("Scale.Range:Minimum"=0.0, "Scale.Range:Maximum"=w570) -> ()  [unwired: 2 in, 2 out]
          n1315 = Equal To 0?(x=w526) -> (x = 0?=w491:bool)
          n1316 = Or(x=w491, y=w519) -> ()  [unwired: 1 out]
          n1317 = property on="Image 4" class="IntGraph (strict)"("X Scale.Range:Maximum"=w568) -> ()  [unwired: 2 in, 2 out]
          n1318 = Equal?(x=u16 2, y=w497) -> (x = y?=w494:bool)
          n1319 = And(x=w494, y="Y-Scale") -> (x .and. y?=w493:bool)
          n1320 = case shown="True" w493 {
            tunnel: [w606 w609] -> w499
            tunnel: ["ImageSlide" u32 0 ("ImageSlide")] -> w498
            frame False {
              n1321 = local read "X-pixels"() -> (w607:sgl)
              n1322 = Decrement(x=w607) -> (x-1=w606:sgl)
            }
            frame True {
              n1323 = local read "Number of frames"() -> (w610:sgl)
              n1324 = local read "Y-lines"() -> (w611:sgl)
              n1325 = Multiply(x=w611, y=w610) -> (x*y=w609:sgl)
            }
          }
          n1326 = case shown="4" w574 {
            tunnel: w498 -> [_ w849 w881 w1053 w1234]
            tunnel: "Play Movie" -> [_ w848 w882 w1055 w1233]
            tunnel: "SlideHorizontal" -> [_ _ _ w1054 w1232]
            tunnel: w566 -> [_ _ w883 w1060 w1231]
            tunnel: w540 -> [_ _ w879 w1058 w1230]
            tunnel: [_ _ w885 w1057 w1229] -> w539
            tunnel: w538 -> [_ _ w880 w1059 w1228]
            tunnel: [_ _ w884 w1056 w1227] -> w537
            tunnel: w499 -> [_ _ w878 _ _]
            tunnel: w487 -> [w845 _ _ w1052 w1226]
            tunnel: w486 -> [w844 _ _ w1051 w1225]
            tunnel: w488 -> [w843 w847 w877 w1050 w1224]
            tunnel: w489 -> [w842 w846 w876 w1049 w1223]
            frame 0, Default {
              n1327 = local write "Image 2"(w842) -> ()
              n1328 = local write "Image 1"(w843) -> ()
              n1329 = local write "Image 3"(w845) -> ()
              n1330 = local write "Image 4"(w844) -> ()
            }
            frame 1 {
              n1331 = case shown="True" w848 {
                tunnel: w849 -> [_ w872]
                tunnel: w847 -> [w851 w868]
                tunnel: w846 -> [w850 w867]
                frame True {
                  n1332 = local read "Number of frames"() -> (w852:sgl)
                  n1333 = while {
                    shift-right: [w863] -> _
                    shift-left: i16 0 ("y") -> [w864]
                    tunnel: w852 -> [w862]
                    tunnel: w851 -> [w855]
                    tunnel: w850 -> [w854]
                    stop <- w860 stop-if-true
                    n1334 = local read "Y-lines"() -> (w857:sgl)
                    n1335 = call "ResetToZeroFOCUS.vi"("UpperLimit"=w862, "Running Index"=w864) -> ("New Index"=w859:i32)
                    n1336 = local read "Play Movie"() -> (w861:bool)
                    n1337 = Multiply(x=w859, y=w857) -> (x*y=w856:sgl)
                    n1338 = local write "ImageSlide"(w859) -> ()
                    n1339 = Not(x=w861) -> (.not. x?=w860:bool)
                    n1340 = Array Subset(array=w855, index (col)=w856, length (col)=w857) -> (w866:u8[][])  [unwired: 2 in]
                    n1341 = Array Subset(array=w854, index (col)=w856, length (col)=w857) -> (w865:u8[][])  [unwired: 2 in]
                    n1342 = Increment(x=w859) -> (x+1=w863:i32)
                    n1343 = local write "Image 2"(w865) -> ()
                    n1344 = local write "Image 1"(w866) -> ()
                    n1345 = Wait Until Next ms Multiple(millisecond multiple="Velocity") -> ()  [unwired: 1 out]
                  }
                }
                frame False {
                  n1346 = local read "Y-lines"() -> (w873:sgl)
                  n1347 = Round To Nearest(number=w872) -> (nearest integer value=w871:u32)
                  n1348 = Multiply(x=w873, y=w871) -> (x*y=w869:sgl)
                  n1349 = local read "Y-lines"() -> (w870:sgl)
                  n1350 = Array Subset(array=w868, index (col)=w869, length (col)=w870) -> (w875:u8[][])  [unwired: 2 in]
                  n1351 = Array Subset(array=w867, index (col)=w869, length (col)=w870) -> (w874:u8[][])  [unwired: 2 in]
                  n1352 = local write "Image 2"(w874) -> ()
                  n1353 = local write "Image 1"(w875) -> ()
                }
              }
            }
            frame 2 {
              n1354 = case shown="False" w882 {
                tunnel: w883 -> [w942 _]
                tunnel: [w937 _] -> w885
                tunnel: [w929 _] -> w884
                tunnel: w880 -> [w905 _]
                tunnel: w879 -> [w904 _]
                tunnel: w881 -> [w903 _]
                tunnel: w878 -> [w888 _]
                tunnel: w877 -> [w887 w1027]
                tunnel: w876 -> [w886 w1026]
                frame False {
                  w956 = 0.0
                  w940 = 0.0 ("Scale.Range:Minimum")
                  n1355 = local read "Reset1"() -> (w914:bool)
                  n1356 = local read "index (row)2"() -> (w900:i32)
                  n1357 = local read "Reset2"() -> (w915:bool)
                  n1358 = local read "index (row)1"() -> (w902:i32)
                  n1359 = local read "Y-lines"() -> (w892:sgl)
                  n1360 = local read "Average1"() -> (w901:i32)
                  n1361 = Subtract(x=w888, y=w901) -> (x-y=w941:sgl)
                  n1362 = local read "Number of frames"() -> (w893:sgl)
                  n1363 = local read "Average2"() -> (w899:i32)
                  n1364 = Subtract(x=w888, y=w899) -> (x-y=w939:sgl)
                  n1365 = local read "X-pixels"() -> (w957:sgl)
                  n1366 = Multiply(x=w892, y=w893) -> (x*y=w891:sgl)
